vi "Average.vi"() -> ()   [LabVIEW 2016]
panel:
  out "average":dbl
  in  "4":dbl
  in  "3":dbl
  in  "2":dbl
  in  "1":dbl
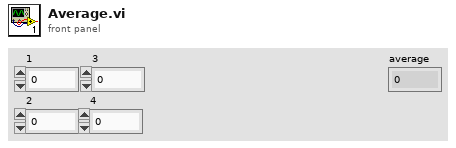
[diagram p1: front panel]
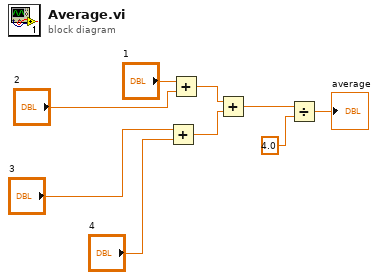
[diagram p0: block diagram]
diagram:
  n1 = Add(x="3", y="4") -> (x+y=w8:dbl)
  n2 = Add(x="1", y="2") -> (x+y=w9:dbl)
  n3 = Add(x=w9, y=w8) -> (x+y=w1:dbl)
  n4 = Divide(x=w1, y=4.0) -> (x/y=→"average":dbl)
